vi "unmarshalling.vi"(7 "Type":variant, 8 "error in (no error)":errorcluster, 10 "B64 Encoded String":string, 11 "Serializer.Base64 in":refnum<class "Serializer.Base64.lvclass">) -> (0 "error out":errorcluster, 2 "Variant":variant, 3 "Serializer.Base64 out":refnum<class "Serializer.Base64.lvclass">)   [LabVIEW 2013, in "Serializer.Base64.lvclass"]
uses:
  Serializer.Base64.lvclass
  <vilib>/LabVIEW Open Source Project/OpenSerializer/Serializer.FlattenedString/Serializer.FlattenedString.lvclass
  <vilib>/LabVIEW Open Source Project/Data Manipulation/TypeDescriptor/OpenDescriptor.lvlib
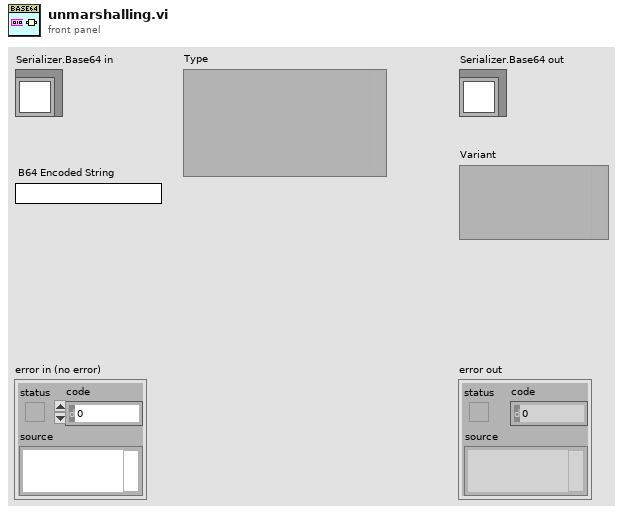
[diagram p1: front panel]
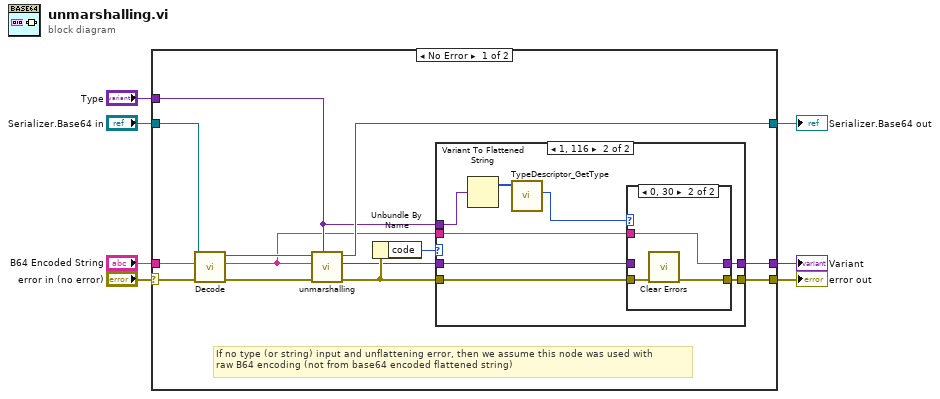
[diagram p0: block diagram]
diagram:
  n1 = case shown="No Error" "error in (no error)" {
    selector: "error in (no error)" -> [w8 w36]
    tunnel: "Serializer.Base64 in" -> [w12 w37]
    tunnel: "B64 Encoded String" -> [w13 _]
    tunnel: [w20 w37] -> w5
    tunnel: [w17 w36] -> w4
    tunnel: [w16 _] -> w3
    tunnel: "Type" -> [w14 _]
    frame No Error {
      # "If no type (or string) input and unflattening error, then we assume this node was used with\nraw B64 encoding (not from base64 encoded flattened string)"
      n2 = call "Decode.vi"("error in (no error)"=w8, "Base64 String"=w13, "Serializer.Base64 in"=w12) -> ("error out"=w9:errorcluster, "decoded string"=w10:string, "Serializer.Base64 out"=w11:refnum<class "Serializer.Base64.lvclass">)  [unwired: 6 in]
      n3 = call-parent "unmarshalling.vi"("Type"=w14, "error in (no error)"=w9, "String"=w10, "Serializer in"=w11) -> ("error out"=w18:errorcluster, "Variant"=w15:variant, "Serializer out"=w20:refnum<class "Serializer.Base64.lvclass">)  [unwired: 5 in]
      n4 = Unbundle By Name(w18) -> ("code"=w19:i32)
      n5 = case shown="1, 116" w19 {
        tunnel: w18 -> [w21 w30]
        tunnel: [w21 w29] -> w17
        tunnel: [w22 w28] -> w16
        tunnel: w15 -> [w22 w27]
        tunnel: w14 -> [_ w25]
        tunnel: w10 -> [_ w26]
        frame Default {
        }
        frame 1, 116 {
          n6 = Variant To Flattened String(Variant=w25) -> (1:w24:i16[])  [unwired: 1 out]
          n7 = call <vilib>:"TypeDescriptor_GetType.vi"("type descriptor"=w24) -> ("Type"=w23:u8)  [unwired: 9 in, 1 out]
          n8 = case shown="0, 30" w23 {
            tunnel: w30 -> [w32 w35]
            tunnel: [w32 w33] -> w29
            tunnel: [w31 w34] -> w28
            tunnel: w27 -> [w31 _]
            tunnel: w26 -> [_ w34]
            frame Default {
            }
            frame 0, 48 {
              n9 = call <vilib>:"Clear Errors.vi"("error in (no error)"=w35) -> ("error out"=w33:errorcluster)  [unwired: 6 in]
            }
          }
        }
      }
    }
    frame Error {
    }
  }
  "error out" <- w4
  "Serializer.Base64 out" <- w5
  "Variant" <- w3
